vi "Main.vi"(8 "error in (no error)":errorcluster) -> (0 "error out":errorcluster, 1 "Canceled?":bool)   [LabVIEW 2015]
panel:
  in  "Numeric":dbl
  out "Waveform Chart":dbl(graph)
  # "Nom de la fenêtre\n\nBref descriptif de comment intéragir avec les éléments graphiques de la fenêtre."
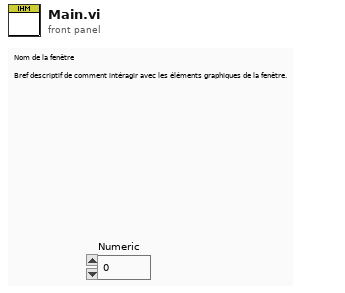
[diagram p1: front panel]
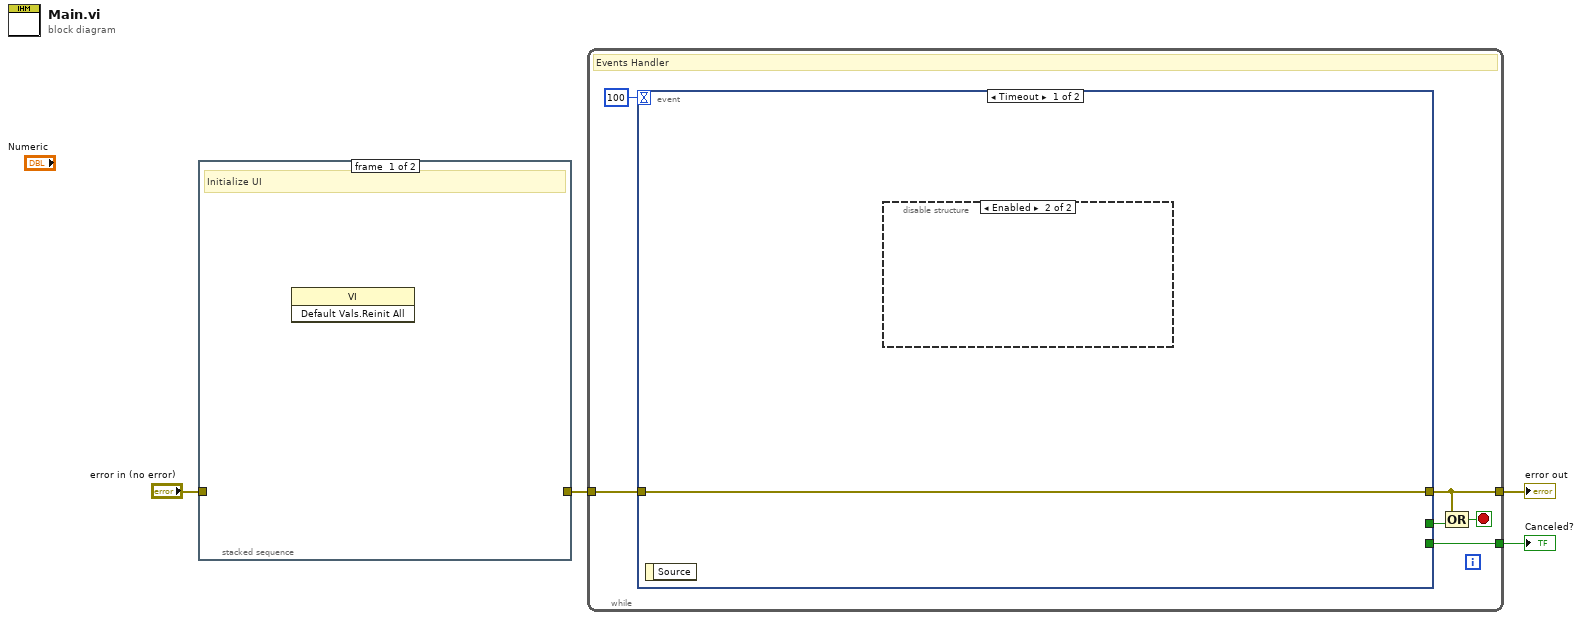
[diagram p0: block diagram]
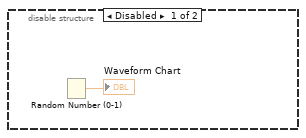
[diagram p2: hidden frame]
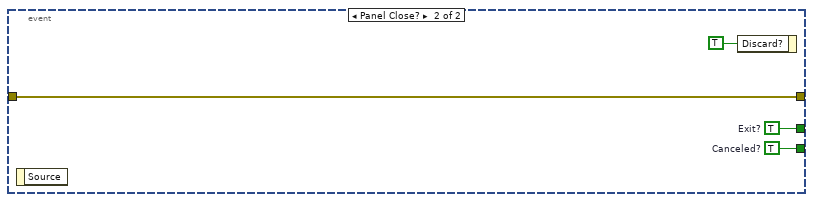
[diagram p3: hidden frame]
diagram:
  n1 = stacked-sequence {
    tunnel: [_ w5] -> w2
    tunnel: "error in (no error)" -> [_ w5]
    frame #0 {
      # "Initialize UI"
      n2 = invoke class="VI" method="Default Vals.Reinit All"() -> ()  [unwired: 3 in, 3 out]
    }
    frame #1 {
      # "Initialize Data"
    }
  }
  n3 = while {
    tunnel: w2 -> [w11]
    tunnel: [w8] -> w4
    tunnel: [w10] -> w3
    stop <- w6 stop-if-true
    # "Events Handler"
    n4 = event shown="[0] Timeout" {
      selector: _ -> [_ _]
      dyn-events: _ -> [_ _]
      timeout: 100 -> [_ _]
      tunnel: [_ w16] -> w7
      tunnel: [w12 w17] -> w8
      tunnel: w11 -> [w12 w17]
      tunnel: [_ w14] -> w10
      event Timeout {
        n5 = event-data() -> ()  [unwired: 1 in, 1 out]
        n6 = disable-structure shown="Enabled" {
          frame Disabled {
            n7 = Random Number (0-1)() -> (number: 0 to 1=→"Waveform Chart":dbl)
          }
          frame Enabled {
          }
        }
      }
      event Panel Close? {
        w14 = TRUE  # Canceled?
        w16 = TRUE  # Exit?
        n8 = event-data() -> ()  [unwired: 1 in, 1 out]
        n9 = event-data("Discard?"=TRUE) -> ()  [unwired: 1 in, 1 out]
      }
    }
    n10 = Compound Arithmetic op=OR(w8, w7) -> (w6:bool)
  }
  "error out" <- w4
  "Canceled?" <- w3
